vi "Create Map from Message Indexes to Tx Write Info.vi"(8 "error in":errorcluster, 9 "1553 channel handles":T1[](array[typedef]) {"terminal status channels" format="%.0x"; "error count channel refs"."wrong sync" format="%.0x"; "error count channel refs"."word" format="%.0x"; "error count channel refs"."unconfigured frames" format="%.0x"; "error count channel refs"."parity" format="%.0x"; "error count channel refs"."monitor" format="%.0x"; "error count channel refs"."Manchester" format="%.0x"; "error count channel refs"."improper number of words" format="%.0x"; "error count channel refs"."general protocol" format="%.0x"; "messages"."Rx status handles" format="%.0x"; "messages"."Tx status handles" format="%.0x"; "messages"."timestamps" format="%.0x"; "messages"."parameters"."RxBC channel handle" format="%.0x"; "messages"."parameters"."RxRT channel handle" format="%.0x"; "messages"."parameters"."Tx channel handle" format="%.0x"}, 10 "hardware handles":T6, 11 "1553 channels":T7[](array[typedef])) -> (0 "error out":errorcluster, 3 "map from message indexes to Tx write info":T13)   [LabVIEW 2020, in "AIM MIL-STD-1553 Engine.lvlib" / "Custom Device.lvlib"]
uses:
  Custom Device.lvlib
  Shared/Map of Message Indexes to Tx Write Info.ctl
  Shared/Tx Write Info.ctl
  Shared/1553 Channel.ctl
  Shared/Address.ctl
  Shared/Message Definition.ctl
  Shared/Message Type.ctl
  Shared/Terminal Endpoint.ctl
  Shared/Parameter Definition.ctl
  Hardware Handles.ctl
  Implementation/Execution Unit/1553 Channel Handles.ctl
  Implementation/Execution Unit/Message Handles.ctl
  Implementation/Execution Unit/Parameter Handles.ctl
  <vilib>/NI VeriStand/Custom Device API/Custom Device Item Ref.ctl
  Shared/Error Count Channel Refs.ctl
  <vilib>/NI VeriStand/Custom Device API/Custom Device API.lvlib
  Implementation/Execution Unit/Execution Unit.lvclass
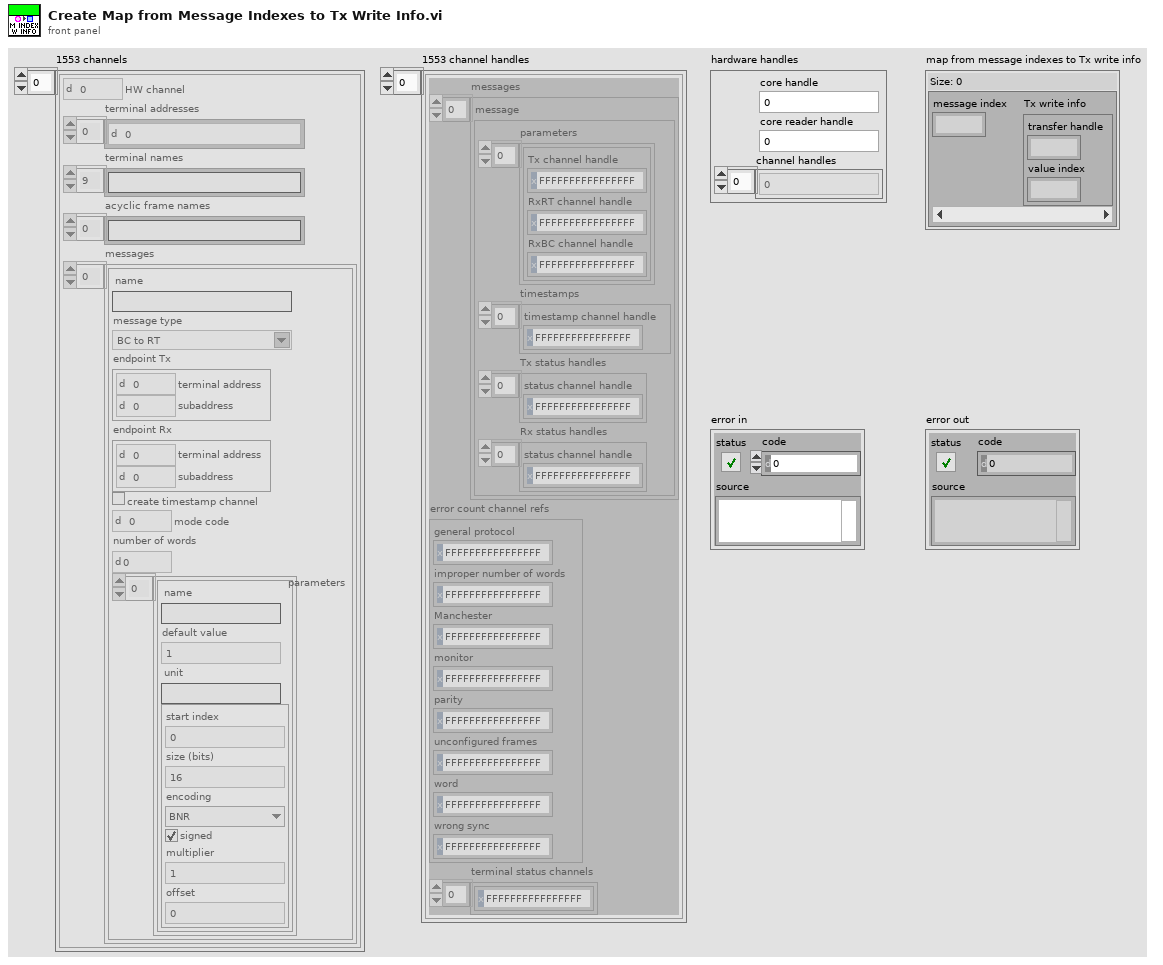
[diagram p1: front panel]
types:
  T1 = typedef "AIM MIL-STD-1553 Engine.lvlib/Implementation.lvlib/Execution Unit.lvclass/1553 Channel Handles.ctl" = cluster{"messages":T2[], "error count channel refs":T5, "terminal status channels":T4[]}
  T2 = typedef "AIM MIL-STD-1553 Engine.lvlib/Implementation.lvlib/Execution Unit.lvclass/Message Handles.ctl" = cluster{"parameters":T3[], "timestamps":T4[], "Tx status handles":T4[], "Rx status handles":T4[]}
  T3 = typedef "AIM MIL-STD-1553 Engine.lvlib/Implementation.lvlib/Execution Unit.lvclass/Parameter Handles.ctl" = cluster{"Tx channel handle":T4, "RxRT channel handle":T4, "RxBC channel handle":T4}
  T4 = typedef "Custom Device API.lvlib/Custom Device Item Ref.ctl" = u64
  T5 = typedef "Error Count Channel Refs.ctl" = cluster{"general protocol":T4, "improper number of words":T4, "Manchester":T4, "monitor":T4, "parity":T4, "unconfigured frames":T4, "word":T4, "wrong sync":T4}
  T6 = typedef "AIM MIL-STD-1553 Engine.lvlib/Custom Device.lvlib/Hardware Handles.ctl" = cluster{"core handle":u64, "core reader handle":u64, "channel handles":u64[]}
  T7 = typedef "1553 Channel.ctl" = cluster{"HW channel":u16, "terminal addresses":T8[], "terminal names":string[], "acyclic frame names":string[], "messages":T9[]}
  T8 = typedef "Address.ctl" = u16
  T9 = typedef "Message Definition.ctl" = cluster{"name":string, "message type":T10, "endpoint Tx":T11, "endpoint Rx":T11, "create timestamp channel":bool, "mode code":u16, "number of words":u16, "parameters":cluster{"name":string, "default value":dbl, "unit":string, "parameter definition":T12}[]}
  T10 = typedef "Message Type.ctl" = string
  T11 = typedef "Terminal Endpoint.ctl" = cluster{"terminal address":T8, "subaddress":T8}
  T12 = typedef "Parameter Definition.ctl" = cluster{"start index":i32, "size (bits)":i32, "encoding":enum16{"BNR", "BCD", "Discrete"}, "signed":bool, "multiplier":dbl, "offset":dbl}
  T13 = typedef "Map of Message Indexes to Tx Write Info.ctl" = map{i32, T14}
  T14 = typedef "Tx Write Info.ctl" = cluster{"transfer handle":u64, "value index":i32}
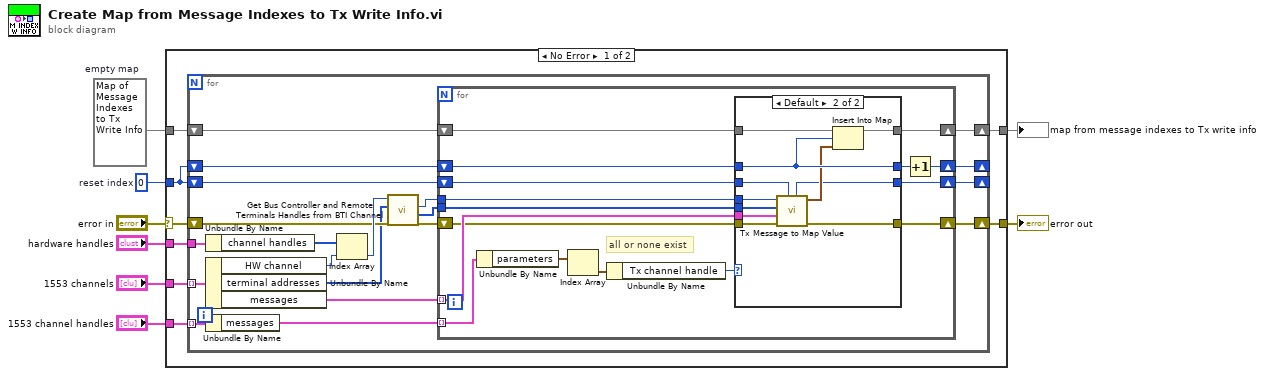
[diagram p0: block diagram]
diagram:
  w1 = 0  # reset index
  w7 = T13 {}  # empty map
  n1 = case shown="No Error" "error in" {
    selector: "error in" -> [w13 w68]
    tunnel: "1553 channels" -> [w10 _]
    tunnel: [w16 w69] -> w2
    tunnel: w7 -> [w15 w69]
    tunnel: "hardware handles" -> [w14 _]
    tunnel: [w12 w68] -> w4
    tunnel: "1553 channel handles" -> [w11 _]
    tunnel: w1 -> [w9 _]
    frame No Error {
      n2 = for {
        tunnel: w10 -> [w36] mode=indexing
        shift-right: [w33] -> w16
        shift-left: w15 -> [w35]
        shift-right: [w31] -> _
        shift-left: w9 -> [w32]
        tunnel: w14 -> [w30]
        shift-right: [w26] -> w12
        shift-left: w13 -> [w22]
        tunnel: w11 -> [w25] mode=indexing
        shift-right: [w20] -> _
        shift-left: w9 -> [w21]
        n3 = Unbundle By Name(w30) -> ("channel handles"=w29:u64[])
        n4 = Unbundle By Name(w36) -> ("HW channel"=w28:u16, "terminal addresses"=w17:T8[], "messages"=w34:T9[])
        n5 = Unbundle By Name(w25) -> ("messages"=w24:T2[])
        n6 = Index Array(array=w29, index=w28) -> (element=w23:u64)
        n7 = call "Get Bus Controller and Remote Terminals Handles from BTI Channel.vi"("error in"=w22, "terminal addresses"=w17, "channel handle in"=w23) -> ("error out"=w27:errorcluster, "remote terminal handles out"=w18:u64[], "bus controller handle out"=w19:u64)  [unwired: 5 in, 1 out]
        n8 = for {
          tunnel: w34 -> [w46] mode=indexing
          shift-right: [w52] -> w33
          shift-left: w35 -> [w51]
          shift-right: [w41] -> w31
          shift-left: w32 -> [w50]
          shift-right: [w48] -> w26
          shift-left: w27 -> [w39]
          tunnel: w18 -> [w47]
          tunnel: w24 -> [w45] mode=indexing
          tunnel: w19 -> [w40]
          shift-right: [w37] -> w20
          shift-left: w21 -> [w38]
          # "all or none exist"
          n9 = Unbundle By Name(w45) -> ("parameters"=w44:T3[])
          n10 = Index Array(array=w44) -> (element=w43:T3)  [unwired: 1 in]
          n11 = Unbundle By Name(w43) -> ("Tx channel handle"=w42:T4)
          n12 = case shown="Default" w42 {
            tunnel: [w56 w67] -> w52
            tunnel: w51 -> [w56 w66]
            tunnel: w50 -> [w55 w65]
            tunnel: [w55 w65] -> w49
            tunnel: w39 -> [w54 w64]
            tunnel: [w54 w63] -> w48
            tunnel: w47 -> [_ w60]
            tunnel: w46 -> [_ w61]
            tunnel: w40 -> [_ w59]
            tunnel: w38 -> [w53 w58]
            tunnel: [w53 w57] -> w37
            frame 0, -1 {
              # "Tx channel handle does not exist for this message, so leave out of the map."
            }
            frame Default {
              n13 = call "Tx Message to Map Value.vi"("parameter index"=w58, "error in"=w64, "message"=w61, "remote terminal handles"=w60, "bus controller handle"=w59) -> ("error out"=w63:errorcluster, "Tx write info"=w62:T14, "next parameter index"=w57:i32)  [unwired: 4 in]
              n14 = Insert Into Map(map in=w66, key=w65, value=w62) -> (map out=w67:T13)  [unwired: 2 out]
            }
          }
          n15 = Increment(x=w49) -> (x+1=w41:i32)
        }
      }
    }
    frame Error {
    }
  }
  "map from message indexes to Tx write info" <- w2
  "error out" <- w4
